vi "FeedbackDecode_VariablesToString_MDArray.vi"(3 "Format":string="%0.2f", 4 "Terminate?":bool=TRUE, 5 "ValueIn":dbl[][](array[numeric]), 6 "FieldName":string, 7 "Type":enum16{"Normal", "Matlab"}(ring)=enum."Matlab") -> (1 "StringOut":string)   [LabVIEW 2020]
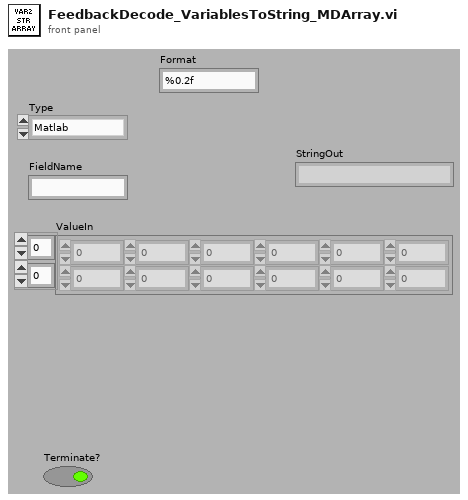
[diagram p1: front panel]
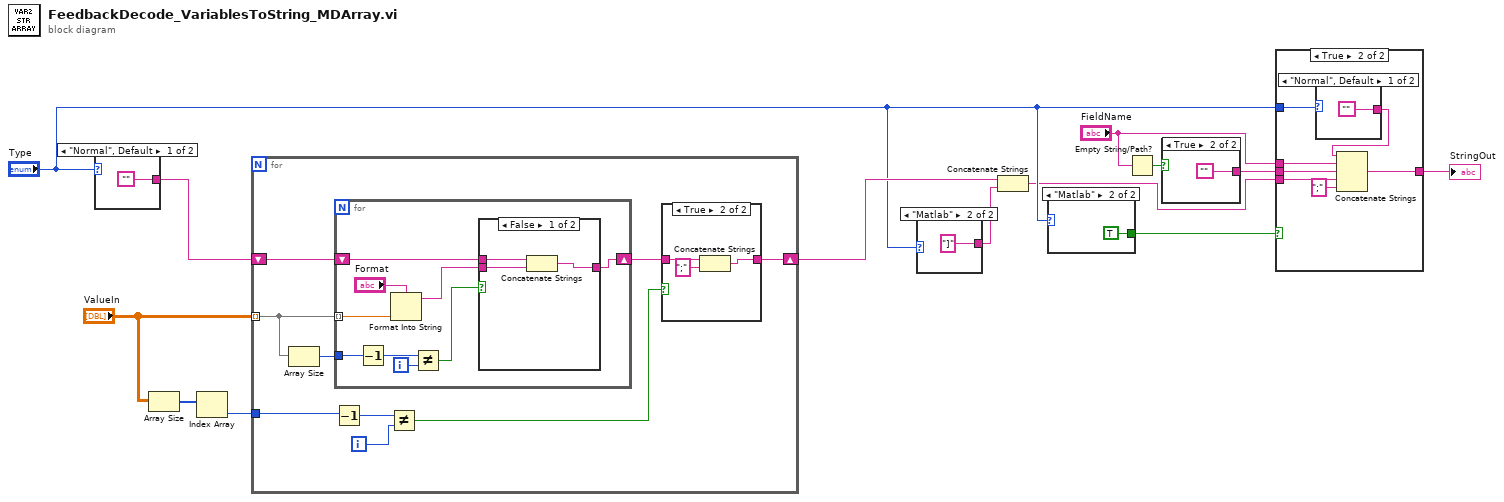
[diagram p0: block diagram]
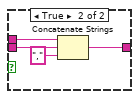
[diagram p3: hidden frame]
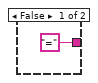
[diagram p4: hidden frame]
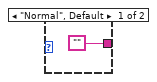
[diagram p5: hidden frame]
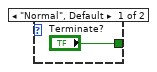
[diagram p6: hidden frame]
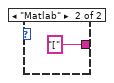
[diagram p7: hidden frame]
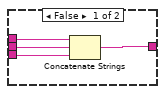
[diagram p8: hidden frame]
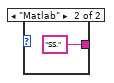
[diagram p9: hidden frame]
diagram:
  n1 = case shown="\"Normal\", Default" "Type" {
    tunnel: ["" "["] -> w13
    frame "Normal", Default {
    }
    frame "Matlab" {
    }
  }
  n2 = Array Size(array="ValueIn") -> (size(s)=w1:i32[])
  n3 = Index Array(array=w1) -> (element=w2:i32)  [unwired: 1 in]
  n4 = for {
    tunnel: "ValueIn" -> [w23] mode=indexing
    shift-right: [w16] -> w9
    shift-left: w13 -> [w22]
    tunnel: w2 -> [w20]
    i -> [w19]
    n5 = Array Size(array=w23) -> (size(s)=w24:i32)
    n6 = Decrement(x=w20) -> (x-1=w21:i32)
    n7 = for {
      tunnel: w23 -> [w37] mode=indexing
      shift-right: [w36] -> w17
      shift-left: w22 -> [w35]
      tunnel: w24 -> [w33]
      i -> [w31]
      n8 = Decrement(x=w33) -> (x-1=w32:i32)
      n9 = Format Into String(format string="Format", w37) -> (resulting string=w34:string)  [unwired: 2 in, 1 out]
      n10 = Not Equal?(x=w32, y=w31) -> (x != y?=w30:bool)
      n11 = case shown="False" w30 {
        tunnel: [w38 w44] -> w36
        tunnel: w35 -> [w40 w43]
        tunnel: w34 -> [w39 w42]
        frame False {
          n12 = Concatenate Strings(w40, w39) -> (w38:string)
        }
        frame True {
          n13 = Concatenate Strings(w43, w42, "," ("string")) -> (w44:string)
        }
      }
    }
    n14 = Not Equal?(x=w21, y=w19) -> (x != y?=w18:bool)
    n15 = case shown="True" w18 {
      tunnel: w17 -> [w25 w28]
      tunnel: [w25 w26] -> w16
      frame False {
      }
      frame True {
        n16 = Concatenate Strings(w28, ";" ("string")) -> (w26:string)
      }
    }
  }
  n17 = case shown="\"Matlab\"" "Type" {
    tunnel: ["" "]"] -> w8
    frame "Normal", Default {
    }
    frame "Matlab" {
    }
  }
  n18 = Concatenate Strings(w9, w8) -> (w6:string)
  n19 = case shown="\"Matlab\"" "Type" {
    tunnel: ["Terminate?" TRUE ("Terminate?")] -> w10
    frame "Normal", Default {
    }
    frame "Matlab" {
    }
  }
  n20 = Empty String/Path?(string/path="FieldName") -> (empty?=w4:bool)
  n21 = case shown="True" w4 {
    tunnel: ["=" ("string") ""] -> w12
    frame False {
    }
    frame True {
    }
  }
  n22 = case shown="True" w10 {
    tunnel: "FieldName" -> [w54 w61]
    tunnel: w12 -> [w53 w60]
    tunnel: w6 -> [w52 w59]
    tunnel: [w51 w57] -> w11
    tunnel: "Type" -> [_ w55]
    frame False {
      n23 = Concatenate Strings(w54, w53, w52) -> (w51:string)
    }
    frame True {
      n24 = case shown="\"Normal\", Default" w55 {
        tunnel: ["" "SS."] -> w56
        frame "Normal", Default {
        }
        frame "Matlab" {
        }
      }
      n25 = Concatenate Strings(w56, w61, w60, w59, ";" ("string")) -> (w57:string)
    }
  }
  "StringOut" <- w11
